vi "Properties Table.vi"(5 "Properties":T1=4211904 items=["SENSOR MODE"=4212128, "CCD MODE"=4212384, "READOUT MODE"=4211872, "ACTIVE VIEW INDEX"=4343136, "BITS PER CHANNEL"=4342976, "IMAGE PIXEL TYPE"=4343296, "BINNING"=4215968, "EXPOSURE TIME"=2049184, "CONTRAST GAIN"=3163312, "CONTRAST OFFSET"=3163328, "LIGHT MODE"=2114720, "SENSITIVITY"=2114992, "PHOTON IMAGING MODE"=2115200, "HIGH DYNAMIC RANGE MODE"=3163360, "WHITE BALANCE"=3163568, "TEMPERATURE"=2115232, "TEMPERATURE TARGET"=2115264, "SENSOR COOLER FAN"=2115296, "LINEBUNDLE HEIGHT"=4212192, "MECHANICAL SHUTTER"=2115488, "BACK FOCUS POSITION"=8422304, "TRIGGER CONNECTOR"=1066432, "TRIGGER SOURCE"=1066144, "OUTPUT TRIGGER SOURCE"=1852576, "TRIGGER GLOBAL EXPOSURE"=2049680, "FIRST TRIGGER BEHAVIOR"=2049696, "CHANNEL SYNC"=1852352, "READOUT DIRECTION"=4211904, "PRE HSYNC COUNT"=1852704, "INTERNAL LINE SPEED"=4191408, "INTERNAL LINE INVERVAL"=4191424], 7 "error in (no error)":errorcluster, 8 "Handle In":u32) -> (0 "Values Out":dbl[](array[numeric]), 1 "Value Stirngs Out":string[](array[string]), 2 "Row Headers":string[](array[string]), 3 "Handle Out":u32, 4 "error out":errorcluster)   [LabVIEW 2015]
uses:
  Camera Properties.ctl
panel:
  in  "Cluster":cluster{"String":string, "Combo Box":string}
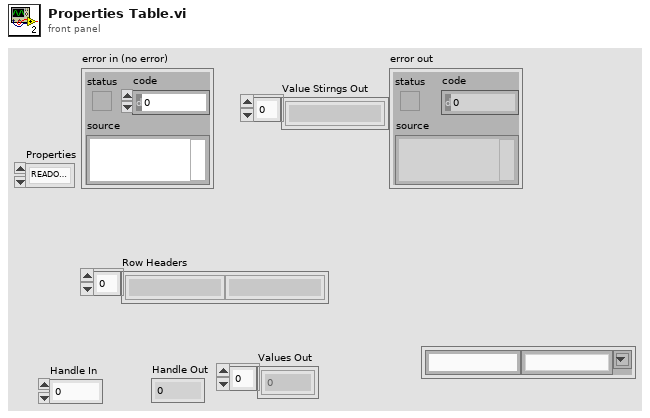
[diagram p1: front panel]
types:
  T1 = typedef "Camera Properties.ctl" = u32
  T2 = typedef "LVStringsAndValuesArrayTypeDef_U32.ctl" = cluster{"String":string, "Value":u32}[]
  T3 = cluster{"Cluster":cluster{"String":string, "Combo Box":string}, "Cluster":cluster{"String":string, "Combo Box":string}}
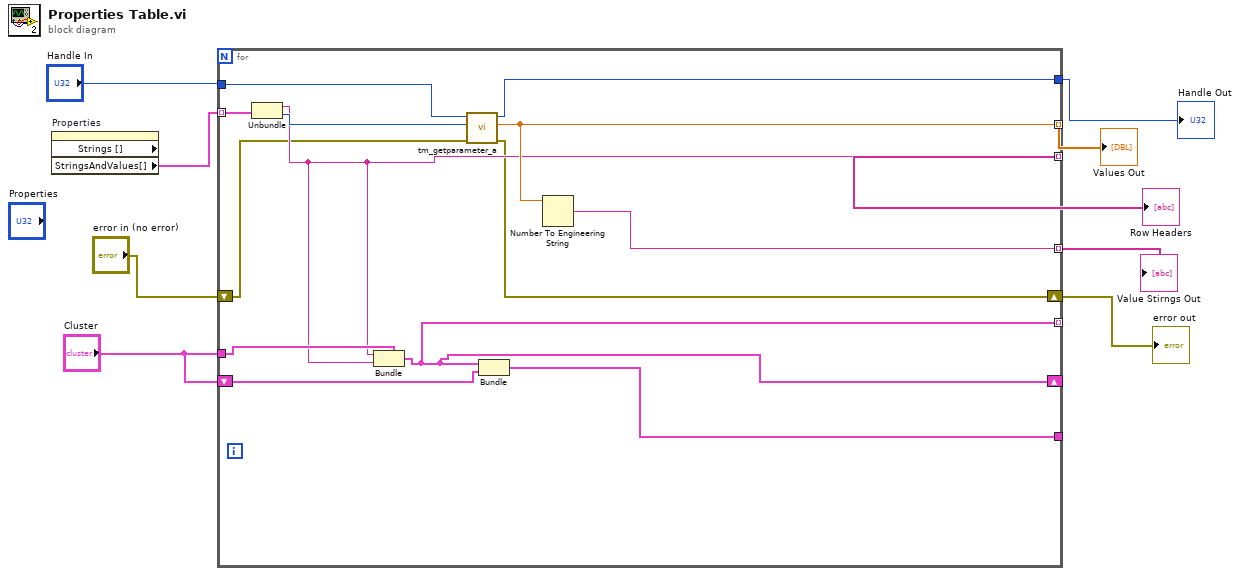
[diagram p0: block diagram]
diagram:
  n1 = property on="Properties" class="Ring (strict)" props=["Strings []", "StringsAndValues[]"]() -> ("StringsAndValues[]"=w4:T2)  [unwired: 2 in, 3 out]
  n2 = for {
    tunnel: w4 -> [w20] mode=indexing
    tunnel: "Handle In" -> [w22]
    tunnel: [w21] -> w8
    tunnel: [w13] -> w7 mode=indexing
    tunnel: [w19] -> w6 mode=indexing
    tunnel: [w18] -> w5 mode=indexing
    tunnel: "Cluster" -> [w15]
    shift-right: [w12] -> _
    shift-left: "Cluster" -> [w16]
    tunnel: [w14] -> _
    tunnel: [w12] -> _ mode=indexing
    shift-right: [w10] -> w1
    shift-left: "error in (no error)" -> [w11]
    n3 = Unbundle(w20) -> ("String"=w13:string, "Value"=w17:u32)
    n4 = Bundle(cluster=w15, "String"=w13, "Combo Box"=w13) -> (w12:cluster{"String":string, "Combo Box":string})
    n5 = call "tm_getparameter_a.vi"("error in (no error)"=w11, "Parameter"=w17, "Handle in"=w22) -> ("error out"=w10:errorcluster, "Value out"=w19:dbl, "Handle out"=w21:u32)  [unwired: 6 in]
    n6 = Bundle("Cluster"=w12, "Cluster"=w16) -> (w14:T3)  [unwired: 1 in]
    n7 = Number To Engineering String(4:w19) -> (0:w18:string)  [unwired: 3 in]
  }
  "Handle Out" <- w8
  "Row Headers" <- w7
  "Values Out" <- w6
  "Value Stirngs Out" <- w5
  "error out" <- w1
